vi "Find Point Correspondences.vi"(7 "Point Correspondence Params (Default: pcl Defaults) in":refnum<class "Point Correspondence Params.lvclass">, 8 "error in (no error)":errorcluster, 10 "Target Points":T2[](array[typedef]), 11 "Source Points":T2[](array[typedef])) -> (0 "error out":errorcluster, 3 "Correspondences":T1[](array[typedef]))   [LabVIEW 2020, in "toolkit.lvlib"]
doc: "Find the correspondences between two unordered 3D Point Sets. This uses the PCL (point cloud library) function pcl::registration::CorrespondenceRejectorSampleConsensus. More details can be found at https://pointclouds.org/documentation/classpcl_1_1registration_1_1_correspondence_rejector_sample_consensus.html"
uses:
  toolkit.lvlib
  Object Point (Float).ctl
  Correspondence Index.ctl
  Point Correspondence Params/Point Correspondence Params.lvclass
  Point Correspondence Params/Point Correspondence Params.lvclass/Point Correspondence Params.ctl
  g_pc_toolkit/bin/gpctoolkit_32-1.dll
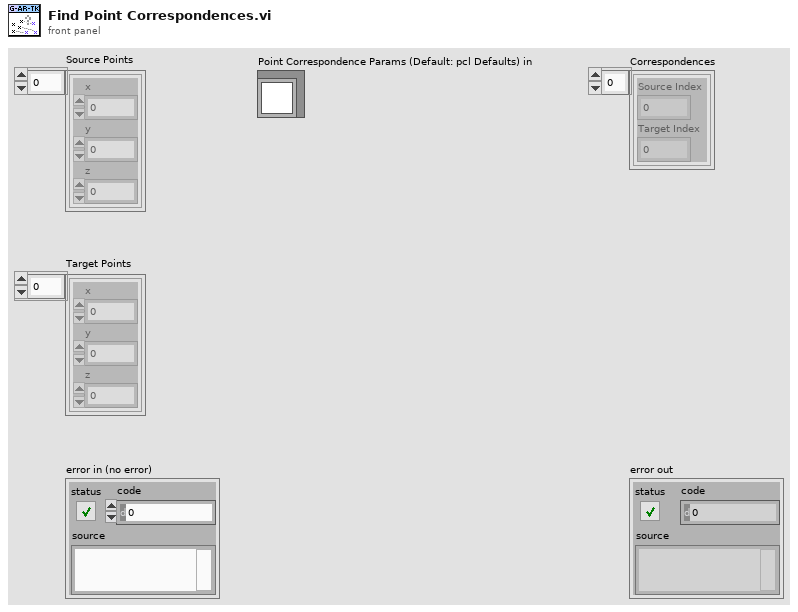
[diagram p1: front panel]
types:
  T1 = typedef "toolkit.lvlib/Correspondence Index.ctl" = cluster{"Source Index":i32, "Target Index":i32}
  T2 = typedef "toolkit.lvlib/Object Point (Float).ctl" = cluster{"x":dbl, "y":dbl, "z":dbl}
  T3 = typedef "toolkit.lvlib/Point Correspondence Params.lvclass/Params.ctl" = cluster{"Refine":bool, "Max Iterations":i32, "Inlier Threshold":dbl}
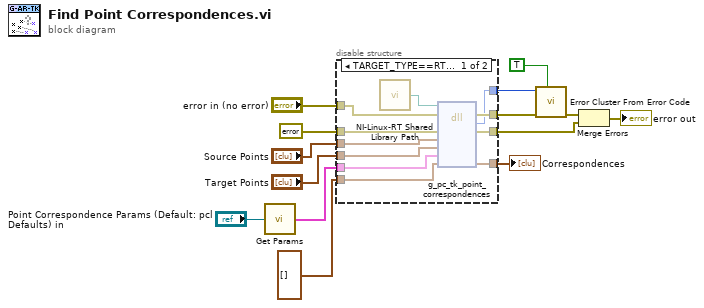
[diagram p0: block diagram]
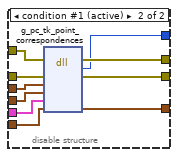
[diagram p2: hidden frame]
diagram:
  n1 = call "Get Params.vi"("Point Correspondence Params in"="Point Correspondence Params (Default: pcl Defaults) in") -> ("Params"=w2:T3)
  n2 = disable-structure shown="TARGET_TYPE==RT&&OS==Linux" {
    disable-tunnel: "error in (no error)" -> [w25 w35]
    disable-tunnel: errorcluster {"status"=FALSE, "code"=0, "source"=""} ("error constant") -> [w21 w31]
    disable-tunnel: [w24 w34] -> w14
    disable-tunnel: [w23 w33] -> w13
    disable-tunnel: [w22 w32] -> w12
    disable-tunnel: "Source Points" -> [w20 w30]
    disable-tunnel: "Target Points" -> [w19 w29]
    disable-tunnel: w2 -> [w18 w28]
    disable-tunnel: T1[] [] -> [w17 w27]
    disable-tunnel: [w16 w26] -> w4
    frame condition #0 {
      n3 = call "NI-Linux-RT Shared Library Path.vi"() -> ("Path"=w15:path)
      n4 = dll-call lib="?" fn="g_pc_tk_point_correspondences" ("g_ar_toolkit.*.*:g_ar_tk_image_copy")(path in=w15, error in=w25, "error_cluster"=w21, "source_points"=w20, "target_points"=w19, "params"=w18, "correspondences"=w17) -> (error out=w24:errorcluster, "MgErr"=w23:i32, "error_cluster"=w22:errorcluster, "correspondences"=w16:T1[])  [unwired: 4 in, 1 out]
    }
    frame condition #1 (active) {
      n5 = dll-call lib="C:/Workspace/CSS/g-point-cloud-toolkit/LabVIEW/g_pc_toolkit/bin/gpctoolkit_*-1.*" fn="g_pc_tk_point_correspondences" ("g_ar_toolkit.*.*:g_ar_tk_image_copy")(error in=w35, "error_cluster"=w31, "source_points"=w30, "target_points"=w29, "params"=w28, "correspondences"=w27) -> (error out=w34:errorcluster, "MgErr"=w33:i32, "error_cluster"=w32:errorcluster, "correspondences"=w26:T1[])  [unwired: 5 in, 1 out]
    }
  }
  "Correspondences" <- w4
  n6 = call <vilib>:"Error Cluster From Error Code.vi"("show call chain? (False)"=TRUE, "error in (no error)"=w14, "error code (0)"=w13) -> ("error out"=w11:errorcluster)  [unwired: 6 in]
  n7 = Merge Errors(w11, w12) -> (→"error out":errorcluster)
